vi "Get Sinks.vi"(8 "error in (no error)":errorcluster, 11 "Registry in":refnum<class "Registry.lvclass">) -> (0 "error out":errorcluster, 2 "Sinks":refnum<class "Sink.lvclass">[](array[class]), 3 "Registry out":refnum<class "Registry.lvclass">)   [LabVIEW 2020, in "LV Log.lvlib" / "Registry.lvclass"]
uses:
  Registry.lvclass
  Sink/Sink.lvclass
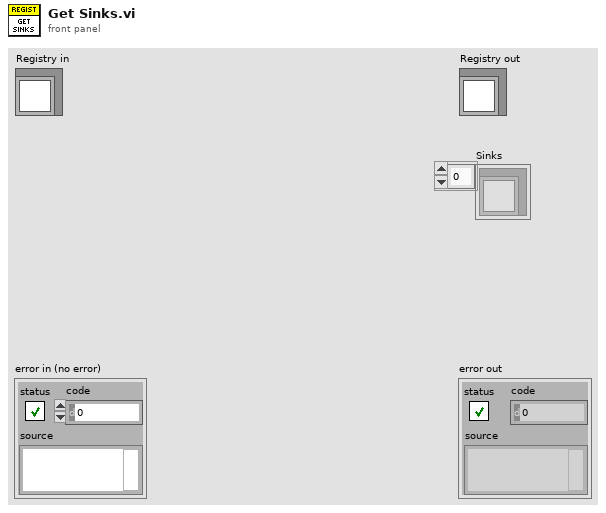
[diagram p1: front panel]
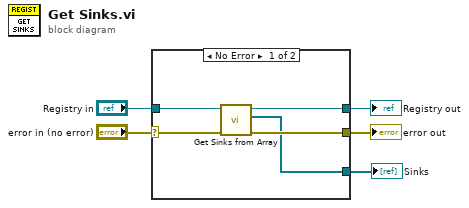
[diagram p0: block diagram]
diagram:
  n1 = case shown="No Error" "error in (no error)" {
    selector: "error in (no error)" -> [w8 w12]
    tunnel: [w7 w12] -> w4
    tunnel: [w9 w11] -> w2
    tunnel: "Registry in" -> [w10 w11]
    tunnel: [w6 _] -> w1
    frame No Error {
      n2 = call "Get Sinks from Array.vi"("error in (no error)"=w8, "Registry in"=w10) -> ("error out"=w7:errorcluster, "Sinks"=w6:refnum<class "Sink.lvclass">[], "Registry out"=w9:refnum<class "Registry.lvclass">)  [unwired: 7 in]
    }
    frame Error {
    }
  }
  "error out" <- w4
  "Registry out" <- w2
  "Sinks" <- w1
